vi "acknowledgeOuterLoopClock.vi"(8 "error in (no error)":errorcluster, 11 "FPGA in":refnum<class "FPGA.lvclass">) -> (0 "error out":errorcluster, 3 "FPGA out":refnum<class "FPGA.lvclass">)   [LabVIEW 2016]
uses:
  FPGA.lvclass
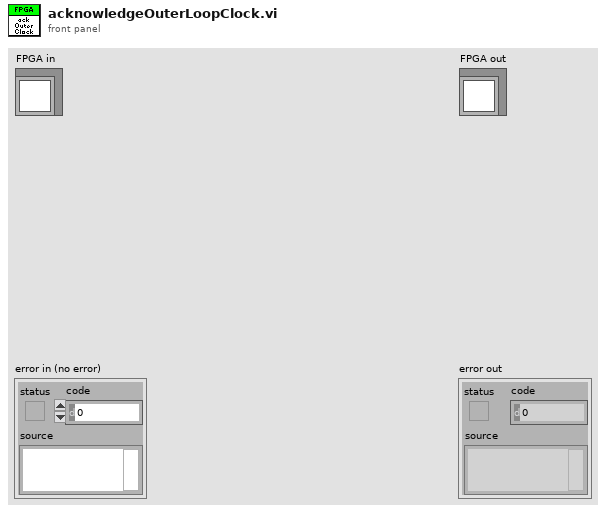
[diagram p1: front panel]
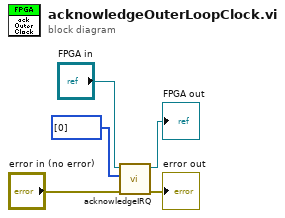
[diagram p0: block diagram]
diagram:
  n1 = call "acknowledgeIRQ.vi"("error in (no error)"="error in (no error)", "IRQs"=i32[] [0], "FPGA in"="FPGA in") -> ("error out"=→"error out":errorcluster, "FPGA out"=→"FPGA out":refnum<class "FPGA.lvclass">)  [unwired: 7 in]
